vi "project.vi"() -> ()   [LabVIEW 2021]
uses:
  <vilib>/addons/Fuzzy Logic/FL Fuzzy Controller (MISO).vi
  <vilib>/addons/Fuzzy Logic/NI_Fuzzy_Logic_API.lvlib
panel:
  out "Right Sensor distance (cm)":dbl format="%#_3g"
  out "Front Sensor distance (cm)":dbl format="%#_3g"
  out "Left Sensor distance (cm)":dbl format="%#_3g"
  out "?":dbl
  out "ARDUINO OUTPUT STRING":string
  out "?":dbl format="%#_2g"
  in  "EMERGENCY STOP":bool
  out "?":dbl format="%#_2g"
  out "Vehicle Speed":dbl(slide) scale=-2.0..3.0
  out "?":bool
  in  "FUZZY SWITCH":bool
  out "TURNING":dbl(knob) scale=-1.0..1.0
  out "?":dbl format="%#_2g"
  out "?":dbl format="%#_2g"
  out "w2, Left wheel angular velocity (rad/s)":dbl format="%#_2g"
  out "w1, Right wheel angular velocity (rad/s)":dbl format="%#_2g"
  in  "Wheel Radius, r (m)":dbl
  in  "Half distance between wheels, L (m)":dbl
  out "Left Wheel RPM":dbl(knob) scale=-20.0..60.0
  out "Right Wheel RPM":dbl(knob) scale=-20.0..60.0
  in  "Vehicle Velocity, v":dbl(slide) scale=-2.0..5.0
  in  "TURNING":dbl(knob) scale=-1.0..1.0
  out "Squirrel Counter":dbl
  out "Vehicle Direction":dbl(knob) scale=0.0..360.0
  out "ASCII Checker":bool
  out "Right Sensor, time (µs)":dbl
  out "Left Sensor, time (µs)":dbl
  out "Front Sensor, time (µs)":dbl
  out "Display of input string":string
  out "Number of characters":dbl
  in  "ARDUINO INPUT STRING":string
  # "ASCII CHARACTER ORDER\n1 - Light Sensor\n2 - Magnetometer\n3 - Left Sensor\n4 - Front Sensor\n5 - Right Sensor"
  # "MANUAL CONTROL"
  # "NORTH"
  # "WEST"
  # "EAST"
  # "SOUTH"
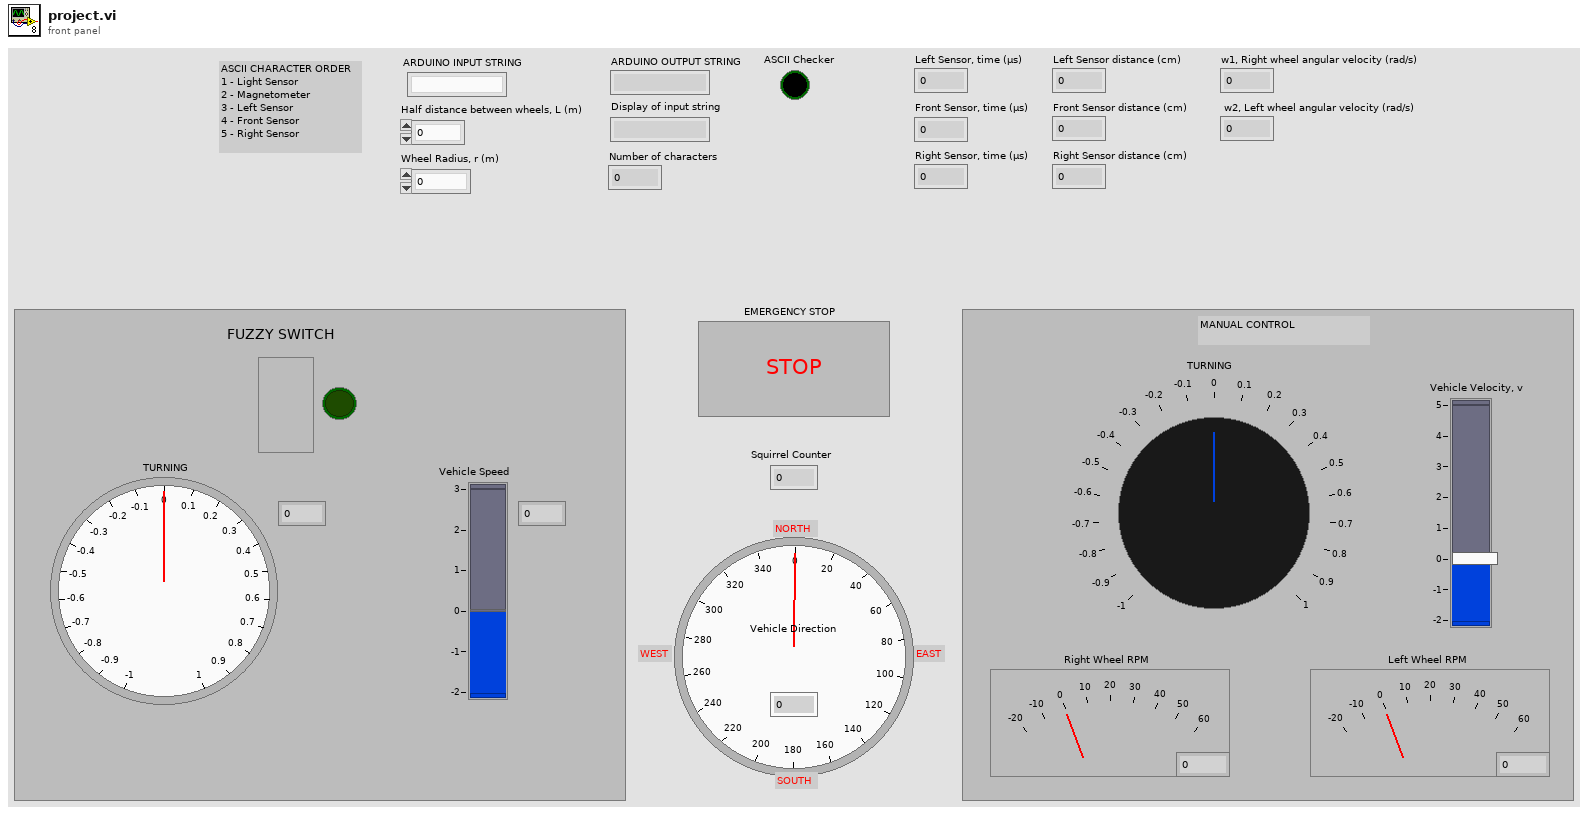
[diagram p1: front panel]
types:
  T1 = typedef "NI_Fuzzy_Logic_API.lvlib/FL System.ctl" = cluster{"input variables":T2[], "output variables":T2[], "rules":T5[], "defuzzification method":T11, "description":string, "user MF interpolating polynomials":T12[]}
  T2 = typedef "NI_Fuzzy_Logic_API.lvlib/FL Variable.ctl" = cluster{"name":string, "range":dbl[], "MFs":T3[]}
  T3 = typedef "NI_Fuzzy_Logic_API.lvlib/FL Membership Function.ctl" = cluster{"name":string, "shape":T4, "points":dbl[], "color":u32, "user-defined shape index":i32}
  T4 = typedef "NI_Fuzzy_Logic_API.lvlib/FL Membership Function Shape.ctl" = u16
  T5 = typedef "NI_Fuzzy_Logic_API.lvlib/FL Rule.ctl" = cluster{"antecedents":T6[], "antecedent connective":T8, "consequents":T9[], "consequent implication":T10, "degree of support":dbl}
  T6 = typedef "NI_Fuzzy_Logic_API.lvlib/FL Antecedent.ctl" = cluster{"Var Index":i32, "MF Index":i32, "Cond":T7}
  T7 = typedef "NI_Fuzzy_Logic_API.lvlib/FL Modifier.ctl" = u16
  T8 = typedef "NI_Fuzzy_Logic_API.lvlib/FL Antecedent Connective.ctl" = u16
  T9 = typedef "NI_Fuzzy_Logic_API.lvlib/FL Consequent.ctl" = cluster{"Var Index":i32, "MF Index":i32, "Cond":T7}
  T10 = typedef "NI_Fuzzy_Logic_API.lvlib/FL Consequent Implication.ctl" = u16
  T11 = typedef "NI_Fuzzy_Logic_API.lvlib/FL Defuzzification.ctl" = u16
  T12 = typedef "NI_Fuzzy_Logic_API.lvlib/FL Interpolating polynomials.ctl" = cluster{"X":dbl[], "Y":dbl[], "Y(x) coeff":dbl[][], "X(y) coeff":dbl[][], "Area(y) coeff":dbl[][], "coa_x(y) coeff":dbl[][]}
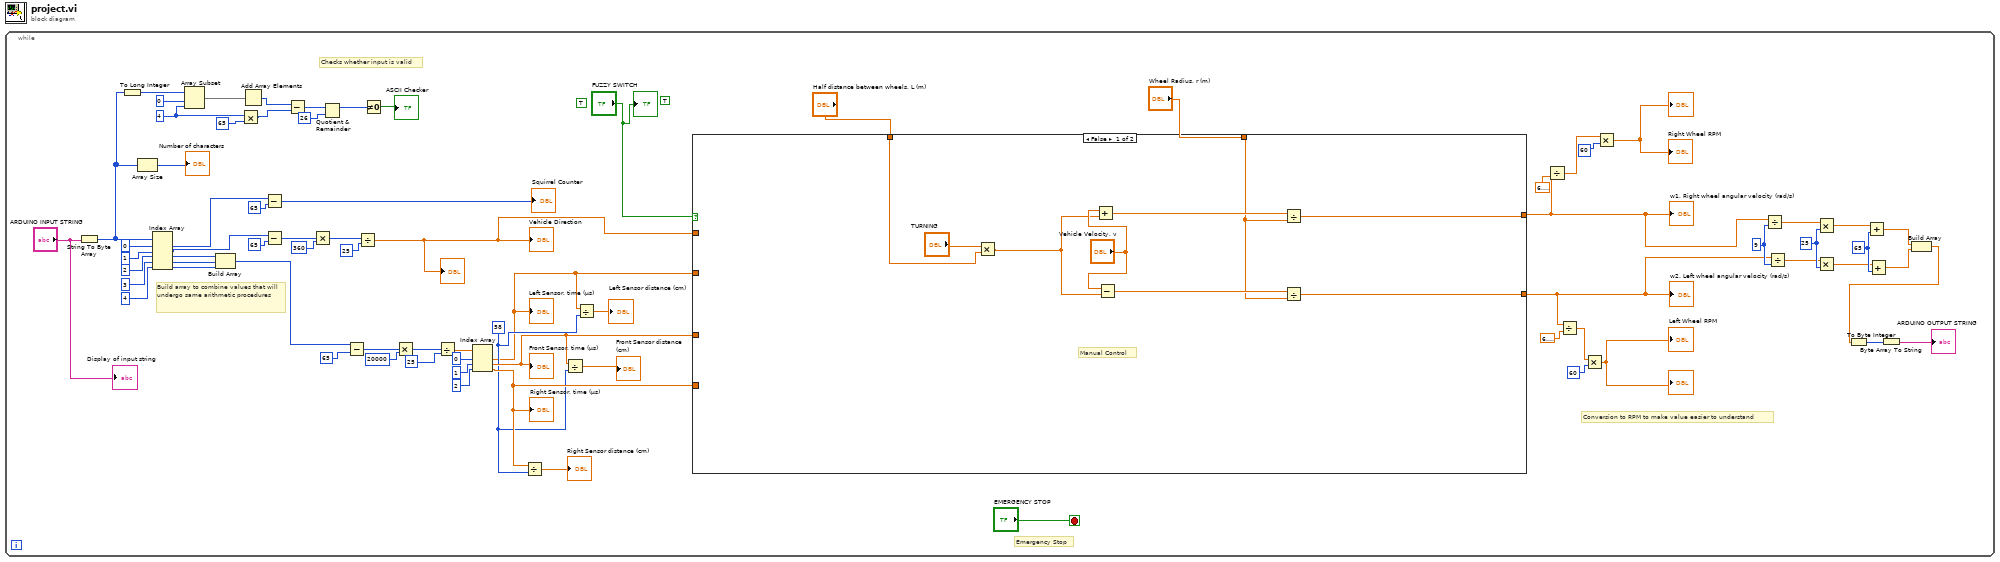
[diagram p0: block diagram]
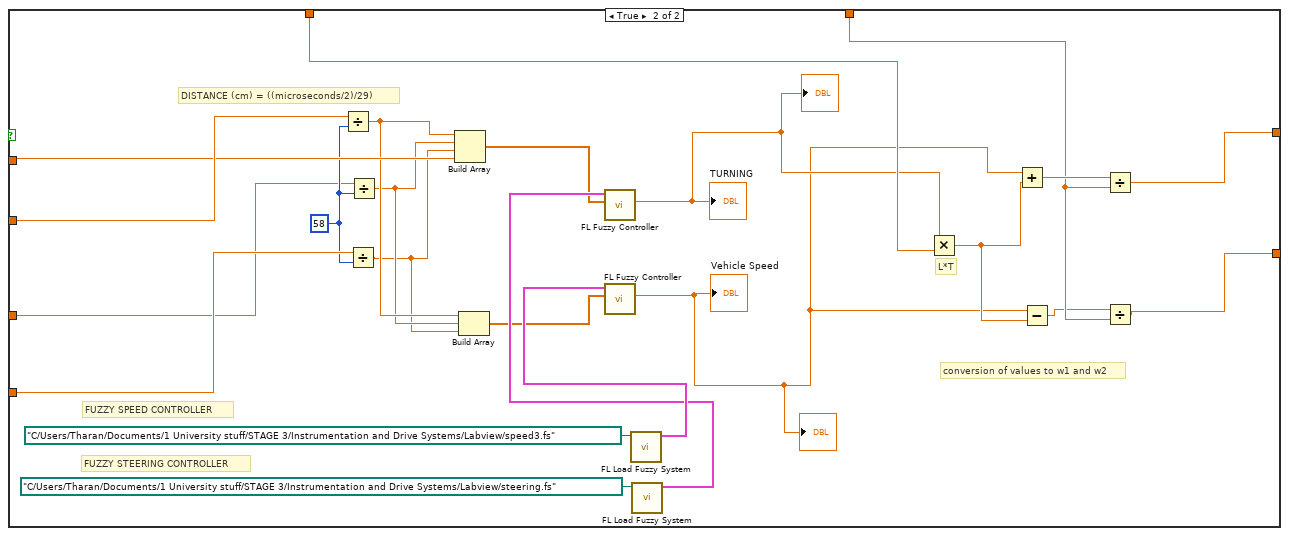
[diagram p2: hidden frame]
diagram:
  n1 = while {
    stop <- "EMERGENCY STOP" stop-if-true
    w3 = 58
    w16 = 65
    w19 = 25
    w21 = 9
    (unwired) TRUE ("FUZZY ON")
    (unwired) TRUE ("FUZZY SWITCH")
    w61 = 4 ("length")
    # "Build array to combine values that will undergo same arithmetic procedures"
    # "Conversion to RPM to make value easier to understand"
    # "Emergency Stop"
    # "Checks whether input is valid"
    n2 = String To Byte Array(string="ARDUINO INPUT STRING") -> (unsigned byte array=w64:u8[])
    n3 = To Long Integer(number=w64) -> (32bit integer=w63:i32[])
    n4 = Array Size(array=w64) -> (size(s)=→"Number of characters":i32)
    n5 = Index Array(array=w64, index #1=0 ("index"), index #2=1 ("index"), index #3=2 ("index"), index #4=3 ("index"), index #5=4 ("index")) -> (element #1=w36:u8, element #2=w42:u8, element #3=w68:u8, element #4=w69:u8, element #5=w70:u8)
    n6 = Array Subset(array=w63, index=0, length=w61) -> (w59:i32[])
    n7 = Build Array(w68, w69, w70) -> (w44:u8[])
    n8 = Multiply(x=w61, y=65) -> (x*y=w57:i32)
    n9 = Add Array Elements(numeric array=w59) -> (sum=w58:i32)
    n10 = Subtract(x=w36, y=65) -> (x-y=→"Squirrel Counter":i32)
    n11 = Subtract(x=w42, y=65) -> (x-y=w40:i32)
    n12 = Subtract(x=w58, y=w57) -> (x-y=w56:i32)
    n13 = Multiply(x=w40, y=360) -> (x*y=w38:i32)
    n14 = Quotient & Remainder(x=w56, y=26) -> (x-y*floor(x/y)=w54:i32)  [unwired: 1 out]
    n15 = Subtract(x=w44, y=u8 65) -> (x-y=w50:u8[])
    n16 = Divide(x=w38, y=25) -> (x/y=w8:dbl)
    "Vehicle Direction" <- w8
    "?" <- w8
    n17 = Not Equal To 0?(x=w54) -> (x != 0?=→"ASCII Checker":bool)
    n18 = Multiply(x=w50, y=20000) -> (x*y=w49:i32[])
    n19 = Divide(x=w49, y=25) -> (x/y=w48:dbl[])
    n20 = Index Array(array=w48, index #1=0 ("index"), index #2=1 ("index"), index #3=2 ("index")) -> (element #1=w2:dbl, element #2=w5:dbl, element #3=w7:dbl)
    "Front Sensor, time (µs)" <- w5
    "Left Sensor, time (µs)" <- w2
    "Right Sensor, time (µs)" <- w7
    n21 = Divide(x=w7, y=w3) -> (x/y=→"Right Sensor distance (cm)":dbl)
    n22 = Divide(x=w5, y=w3) -> (x/y=→"Front Sensor distance (cm)":dbl)
    n23 = Divide(x=w2, y=w3) -> (x/y=→"Left Sensor distance (cm)":dbl)
    n24 = case shown="False" "FUZZY SWITCH" {
      tunnel: "Half distance between wheels, L (m)" -> [w83 w93]
      tunnel: "Wheel Radius, r (m)" -> [w80 w87]
      tunnel: [w79 w88] -> w22
      tunnel: [w78 w85] -> w20
      tunnel: w2 -> [_ w107]
      tunnel: w5 -> [_ w97]
      tunnel: w7 -> [_ w106]
      tunnel: w8 -> [_ w102]
      frame False {
        # "Manual Control"
        n25 = Multiply(x="TURNING", y=w83) -> (x*y=w76:dbl)
        n26 = Add(x="Vehicle Velocity, v", y=w76) -> (x+y=w82:dbl)
        n27 = Subtract(x="Vehicle Velocity, v", y=w76) -> (x-y=w81:dbl)
        n28 = Divide(x=w82, y=w80) -> (x/y=w79:dbl)
        n29 = Divide(x=w81, y=w80) -> (x/y=w78:dbl)
      }
      frame True {
        w98 = 58
        # "conversion of values to w1 and w2"
        # "L*T"
        # "FUZZY STEERING CONTROLLER"
        # "FUZZY SPEED CONTROLLER"
        # "DISTANCE (cm) = ((microseconds/2)/29)"
        n30 = Divide(x=w107, y=w98) -> (x/y=w96:dbl)
        n31 = Divide(x=w106, y=w98) -> (x/y=w94:dbl)
        n32 = Divide(x=w97, y=w98) -> (x/y=w95:dbl)
        n33 = Build Array(w96, w95, w94, w102) -> (w101:dbl[])
        n34 = Build Array(w96, w95, w94) -> (w100:dbl[])
        n35 = call <vilib>:"FL Load Fuzzy System.vi"("file path"=path "C:/Users/Tharan/Documents/1 University stuff/STAGE 3/Instrumentation and Drive Systems/Labview/speed3.fs") -> ("fuzzy system out"=w104:T1)  [unwired: 9 in, 1 out]
        n36 = call-poly <vilib>:"FL Fuzzy Controller.vi"("input values"=w100, "fuzzy system in"=w104) -> ("output value"=w90:dbl)  [unwired: 5 in, 4 out]
        "Vehicle Speed" <- w90
        "?" <- w90
        n37 = call <vilib>:"FL Load Fuzzy System.vi"("file path"=path "C:/Users/Tharan/Documents/1 University stuff/STAGE 3/Instrumentation and Drive Systems/Labview/steering.fs") -> ("fuzzy system out"=w103:T1)  [unwired: 9 in, 1 out]
        n38 = call-poly <vilib>:"FL Fuzzy Controller.vi"("input values"=w101, "fuzzy system in"=w103) -> ("output value"=w92:dbl)  [unwired: 5 in, 4 out]
        "TURNING" <- w92
        "?" <- w92
        n39 = Multiply(x=w92, y=w93) -> (x*y=w91:dbl)
        n40 = Add(x=w90, y=w91) -> (x+y=w89:dbl)
        n41 = Subtract(x=w90, y=w91) -> (x-y=w86:dbl)
        n42 = Divide(x=w89, y=w87) -> (x/y=w88:dbl)
        n43 = Divide(x=w86, y=w87) -> (x/y=w85:dbl)
      }
    }
    "w1, Right wheel angular velocity (rad/s)" <- w22
    "w2, Left wheel angular velocity (rad/s)" <- w20
    n44 = Divide(x=w22, y=6.283185307179586) -> (x/y=w27:dbl)
    n45 = Divide(x=w20, y=6.283185307179586) -> (x/y=w31:dbl)
    n46 = Multiply(x=w31, y=60) -> (x*y=→"Left Wheel RPM" →"?":dbl)
    n47 = Multiply(x=w27, y=60) -> (x*y=→"Right Wheel RPM" →"?":dbl)
    n48 = Divide(x=w22, y=w21) -> (x/y=w18:dbl)
    n49 = Divide(x=w20, y=w21) -> (x/y=w17:dbl)
    n50 = Multiply(x=w18, y=w19) -> (x*y=w15:dbl)
    n51 = Multiply(x=w17, y=w19) -> (x*y=w14:dbl)
    n52 = Add(x=w15, y=w16) -> (x+y=w13:dbl)
    n53 = Add(x=w14, y=w16) -> (x+y=w12:dbl)
    n54 = Build Array(w13, w12) -> (w11:dbl[])
    n55 = To Byte Integer(number=w11) -> (8bit integer=w10:i8[])
    n56 = Byte Array To String(unsigned byte array=w10) -> (string=→"ARDUINO OUTPUT STRING":string)
    "Display of input string" <- "ARDUINO INPUT STRING"
    "?" <- "FUZZY SWITCH"
  }
